vi "ConvertF-V.vi"(6 "Test Name":string(combo)="WDW", 8 "Tolerance":dbl, 11 "Force  Spect":dbl) -> (1 "F-V Lower":dbl format="%#_13g", 2 "F-V Normal":dbl format="%#_13g", 3 "F-V Upper":dbl format="%#_13g")   [LabVIEW 2017]
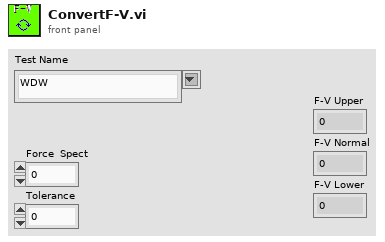
[diagram p1: front panel]
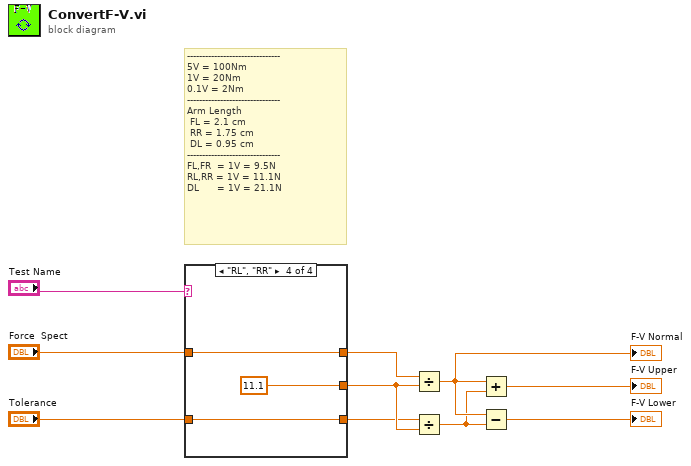
[diagram p0: block diagram]
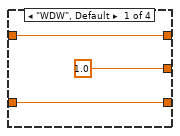
[diagram p2: hidden frame]
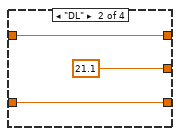
[diagram p3: hidden frame]
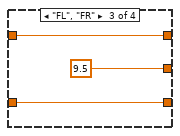
[diagram p4: hidden frame]
diagram:
  # "-------------------------------\n5V = 100Nm\n1V = 20Nm\n0.1V = 2Nm\n-------------------------------\nArm Length\n FL = 2.1 cm\n RR = 1.75 cm\n DL = 0.95 cm\n-------------------------------\nFL,FR  = 1V = 9.5N\nRL,RR = 1V = 11.1N\nDL      = 1V = 21.1N"
  n1 = case shown="\"RL\", \"RR\"" "Test Name" {
    tunnel: "Force  Spect" -> [w13 w14 w19 w22]
    tunnel: "Tolerance" -> [w12 w15 w18 w21]
    tunnel: [1.0 ("y") 21.1 ("y") 9.5 ("y") 11.1 ("y")] -> w5
    tunnel: [w12 w15 w18 w21] -> w4
    tunnel: [w13 w14 w19 w22] -> w3
    frame "WDW", Default {
    }
    frame "DL" {
    }
    frame "FL", "FR" {
    }
    frame "RL", "RR" {
    }
  }
  n2 = Divide(x=w3, y=w5) -> (x/y=w7:dbl)
  "F-V Normal" <- w7
  n3 = Divide(x=w4, y=w5) -> (x/y=w6:dbl)
  n4 = Add(x=w7, y=w6) -> (x+y=→"F-V Upper":dbl)
  n5 = Subtract(x=w7, y=w6) -> (x-y=→"F-V Lower":dbl)
